vi "QuitOnLastWindowClosed-Set.vi"(8 "error in (no error)":errorcluster, 10 "Quit On Last Window Closed":bool, 11 "Engine in":refnum<class "Engine.lvclass">) -> (0 "error out":errorcluster, 3 "Engine out":refnum<class "Engine.lvclass">)   [LabVIEW 2024, in "GLF.lvlib" / "Engine.lvclass"]
uses:
  Engine.lvclass
  Engine.lvclass/Engine.ctl
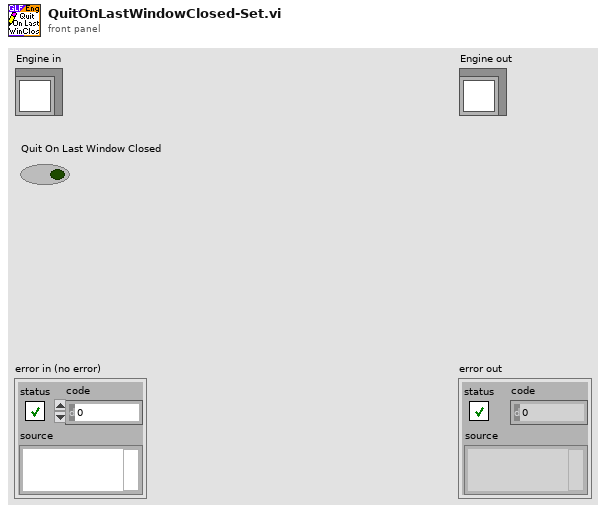
[diagram p1: front panel]
types:
  T1 = typedef "GLF.lvlib/Engine.lvclass/DVR--cluster.ctl" = cluster{"CMD Queue":T2, "Config":T3, "Ctxt":T5, "Metrics":T6}
  T2 = typedef "GLF.lvlib/Engine.lvclass/Command--queue.ctl" = refnum<queue>
  T3 = typedef "GLF.lvlib/Engine.lvclass/Config--cluster.ctl" = cluster{"Quit On Last Window Closed":bool, "VSync":T4, "FPS Target":dbl}
  T4 = typedef "GLF.lvlib/Engine.lvclass/VSync--enum.ctl" = enum16{"Disabled", "Enabled", "Adaptative"}
  T5 = typedef "GLF.lvlib/Engine.lvclass/Context--cluster.ctl" = cluster{"Ticks Begin":u64, "VSync Enabled":bool}
  T6 = typedef "GLF.lvlib/Engine.lvclass/Metrics--cluster.ctl" = cluster{"Uptime [ms]":u64, "Loop Time [ms]":u64}
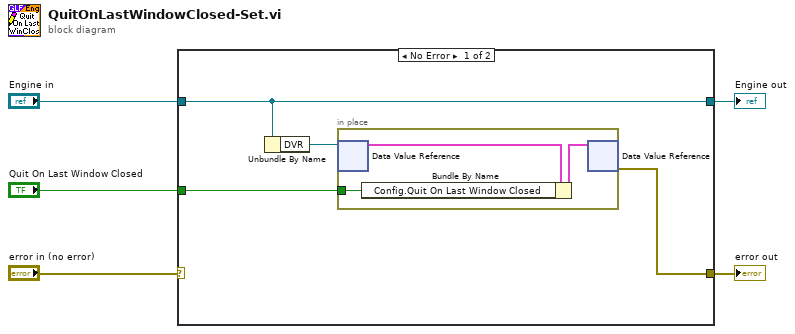
[diagram p0: block diagram]
diagram:
  n1 = case shown="No Error" "error in (no error)" {
    selector: "error in (no error)" -> [_ w13]
    tunnel: [w6 w13] -> w4
    tunnel: [w8 w14] -> w2
    tunnel: "Engine in" -> [w8 w14]
    tunnel: "Quit On Last Window Closed" -> [w7 _]
    frame No Error {
      n2 = Unbundle By Name(w8) -> ("DVR"=w9:refnum<data-value>)
      n3 = in-place {
        in-place-border: w7 -> [w10]
        n4 = in-place-dvr #1(w9) -> (w12:T1)  [unwired: 1 out]
        n5 = Bundle By Name(cluster=w12, "Config.Quit On Last Window Closed"=w10) -> (w11:T1)
        n6 = in-place-dvr #1(w11) -> (w6:errorcluster)  [unwired: 1 out]
      }
    }
    frame Error {
    }
  }
  "error out" <- w4
  "Engine out" <- w2
